vi "VisionBinCoordinates.vi"(3 "Distance to Bin":dbl=nan, 5 "Vision Array Name":string="VisionTable/VisionArray") -> (0 "x Coordinate of Bin":dbl, 1 "bin angle":dbl, 2 "y Coordinate of Bin":dbl)   [LabVIEW 2014]
uses:
  <vilib>/Rock Robotics/Network Tables/NT Read Number.vi
  Robot Global Data.vi
  <vilib>/Rock Robotics/Network Tables/NT Read Numeric Array.vi
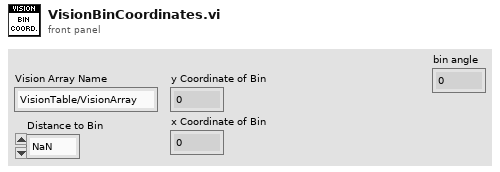
[diagram p1: front panel]
types:
  T1 = cluster{"[0]":dbl, "[1]":dbl, "[2]":dbl, "[3]":dbl, "[4]":dbl, "[5]":dbl, "[6]":dbl, "[7]":dbl, "[8]":dbl, "[9]":dbl, "[10]":dbl, "[11]":dbl}
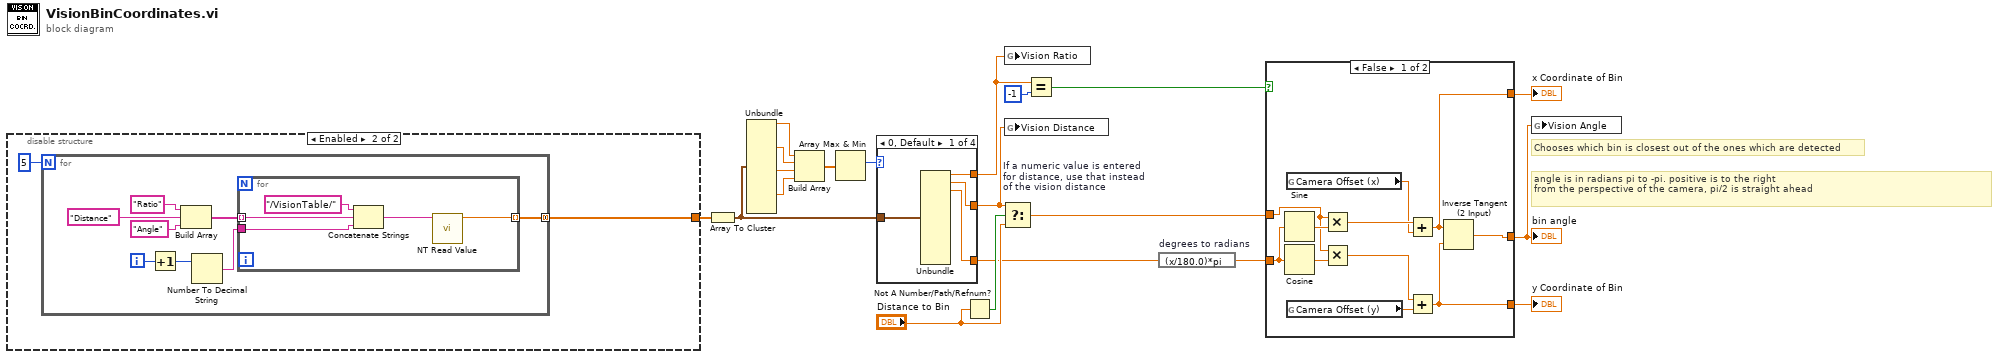
[diagram p0: block diagram]
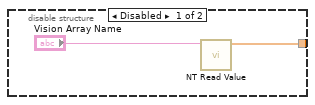
[diagram p2: hidden frame]
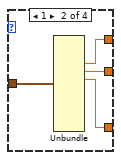
[diagram p3: hidden frame]
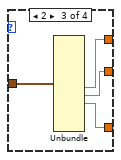
[diagram p4: hidden frame]
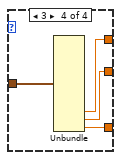
[diagram p5: hidden frame]
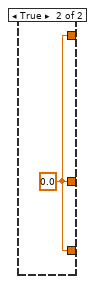
[diagram p6: hidden frame]
diagram:
  # "angle is in radians pi to -pi. positive is to the right \nfrom the perspective of the camera, pi/2 is straight ahead"
  # "Chooses which bin is closest out of the ones which are detected"
  n1 = disable-structure shown="Enabled" {
    disable-tunnel: [w21 w24] -> w20
    frame Disabled {
      n2 = call-poly <vilib>:"NT Read Value.vi"("Name"="Vision Array Name") -> ("Numeric Array"=w21:dbl[])  [unwired: 9 in, 1 out]
    }
    frame Enabled {
      n3 = for {
        N: 5 -> [_]
        tunnel: [w32] -> w24 mode=concatenating
        i -> [w27]
        n4 = Increment(x=w27) -> (x+1=w26:i32)
        n5 = Build Array("Ratio" ("element"), "Distance" ("element"), "Angle") -> (w28:string[])
        n6 = Number To Decimal String(number=w26) -> (decimal integer string=w25:string)  [unwired: 1 in]
        n7 = for {
          tunnel: [w36] -> w32 mode=indexing
          tunnel: w28 -> [w35] mode=indexing
          tunnel: w25 -> [w33]
          n8 = Concatenate Strings("/VisionTable/" ("string"), w35, w33) -> (w37:string)
          n9 = call-poly <vilib>:"NT Read Value.vi"("Name"=w37) -> ("Numeric"=w36:dbl)  [unwired: 9 in, 1 out]
        }
      }
    }
  }
  n10 = Array To Cluster(array=w20) -> (cluster=w16:T1)
  n11 = Unbundle(w16) -> ("[0]"=w4:dbl, "[3]"=w3:dbl, "[6]"=w2:dbl, "[9]"=w1:dbl)  [unwired: 8 out]
  n12 = Build Array(w4, w3, w2, w1) -> (w17:dbl[])
  n13 = Array Max & Min(array=w17) -> (max index (indices)=w5:i32)  [unwired: 3 out]
  n14 = case shown="0, Default" w5 {
    tunnel: w16 -> [w41 w45 w49 w53]
    tunnel: [w40 w44 w48 w52] -> w15
    tunnel: [w39 w42 w46 w50] -> w7
    tunnel: [w38 w43 w47 w51] -> w13
    frame 0, Default {
      n15 = Unbundle(w41) -> ("[0]"=w40:dbl, "[1]"=w38:dbl, "[2]"=w39:dbl)  [unwired: 9 out]
    }
    frame 1 {
      n16 = Unbundle(w45) -> ("[3]"=w44:dbl, "[4]"=w43:dbl, "[5]"=w42:dbl)  [unwired: 9 out]
    }
    frame 2 {
      n17 = Unbundle(w49) -> ("[6]"=w48:dbl, "[7]"=w47:dbl, "[8]"=w46:dbl)  [unwired: 9 out]
    }
    frame 3 {
      n18 = Unbundle(w53) -> ("[9]"=w52:dbl, "[10]"=w51:dbl, "[11]"=w50:dbl)  [unwired: 9 out]
    }
  }
  n19 = Not A Number/Path/Refnum?(number/path/refnum="Distance to Bin") -> (NaN/Path/Refnum?=w14:bool)
  n20 = Select "If a numeric value is entered\nfor distance, use that instead\nof the vision distance"(t=w13, s=w14, f="Distance to Bin") -> (s? t:f=w11:dbl)
  n21 = global write "Robot Global Data.vi" "Vision Ratio"(w15) -> ()
  n22 = global write "Robot Global Data.vi" "Vision Distance"(w13) -> ()
  n23 = Equal?(x=w15, y=-1) -> (x = y?=w18:bool)
  n24 = expression code="(x/180.0)*pi" "degrees to radians"(w7) -> (w8:dbl)
  n25 = case shown="False" w18 {
    tunnel: w8 -> [w60 _]
    tunnel: w11 -> [w62 _]
    tunnel: [w55 w65] -> w10
    tunnel: [w54 w65] -> w9
    tunnel: [w56 w65] -> w6
    frame False {
      n26 = Sine(x=w60) -> (sin(x)=w63:dbl)
      n27 = Cosine(x=w60) -> (cos(x)=w64:dbl)
      n28 = global read "Robot Global Data.vi" "Camera Offset (x)"() -> (w59:dbl)
      n29 = global read "Robot Global Data.vi" "Camera Offset (y)"() -> (w57:dbl)
      n30 = Multiply(x=w62, y=w63) -> (x*y=w61:dbl)
      n31 = Multiply(x=w62, y=w64) -> (x*y=w58:dbl)
      n32 = Add(x=w61, y=w59) -> (x+y=w54:dbl)
      n33 = Add(x=w58, y=w57) -> (x+y=w55:dbl)
      n34 = Inverse Tangent (2 Input)(1:w55, 2:w54) -> (0:w56:dbl)
    }
    frame True {
      w65 = 0.0
    }
  }
  "y Coordinate of Bin" <- w10
  "x Coordinate of Bin" <- w9
  "bin angle" <- w6
  n35 = global write "Robot Global Data.vi" "Vision Angle"(w6) -> ()
